vi "Read U8 From 1 Address.vi"(8 "error in (no error)":errorcluster, 9 "Address number (0)":u8 max=49, 10 "Motor ID (0)":u8, 11 "Dynamixel Motor in":refnum<class "Dynamixel Motor.lvclass">) -> (0 "error out":errorcluster, 2 "Data":u8, 3 "Dynamixel Motor out":refnum<class "Dynamixel Motor.lvclass">)   [LabVIEW 2016, in "Dynamixel Motor.lvclass"]
doc: "Reads a single value/address from the motor's register. This is a Low-Level VI that is used by other VIs."
uses:
  <instrlib>/Dynamixel Motor/HAIOL/Dynamixel Motor.lvclass
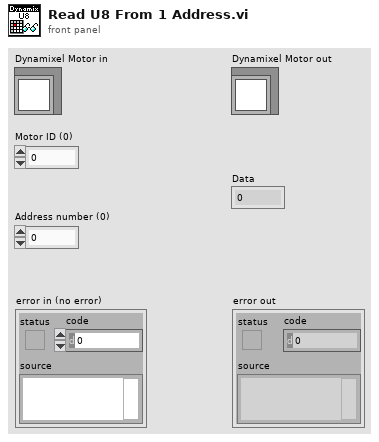
[diagram p1: front panel]
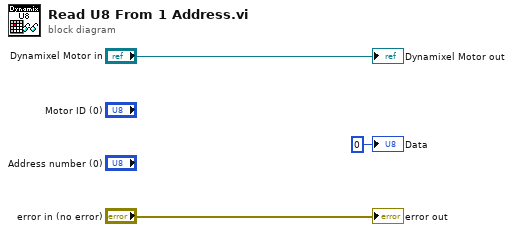
[diagram p0: block diagram]
diagram:
  "error out" <- "error in (no error)"
  "Dynamixel Motor out" <- "Dynamixel Motor in"
  "Data" <- u8 0 ("Data")
